vi "UI.vi"(11 "Error In":errorcluster) -> (15 "Error Out":errorcluster)   [LabVIEW 2020, in "I2C Controller.lvlib" / "I2C.lvclass"]
uses:
  I2C.lvclass
  Typedef's/I2C Timings.ctl
  Typedef's/I2C Operations.ctl
  Common/Typedef's/Protocols Queue Operations.ctl
  Common/Typedef's/Protocols Queue State.ctl
  Common/Typedef's/Protocols Event Operations.ctl
  Typedef's/I2C Data Cluster.ctl
  Parent/Protocols/Protocols.lvclass
  Parent/Protocols/Typedef's/DVR Operations.ctl
  I2C.lvclass/I2C.ctl
  I2C Controller.lvlib
panel:
  in  "Data":u8 format="%x"
  in  "Register Address":u8 format="%x"
  in  "Device Address":u8 format="%x"
  in  "Ok":bool
  in  "Operation":T1
  in  "Timings":T2={"T hd:sta"=4000, "T su:dat"=0, "T hd:dat"=0, "T low"=0, "T high"=0, "T su:sta"=5000, "T su:sto"=5000, "T buf"=5000} {"T buf" step=1 format="%#_6f"; "T su:sto" step=1 format="%#_6f"; "T su:sta" step=1 format="%#_6f"; "T high" step=1 format="%#_6f"; "T low" step=1 format="%#_6f"; "T hd:dat" step=1 format="%#_6f"; "T su:dat" step=1 format="%#_6f"; "T hd:sta" step=1 format="%#_6f"}
  # "All init values is\nfor 100khz"
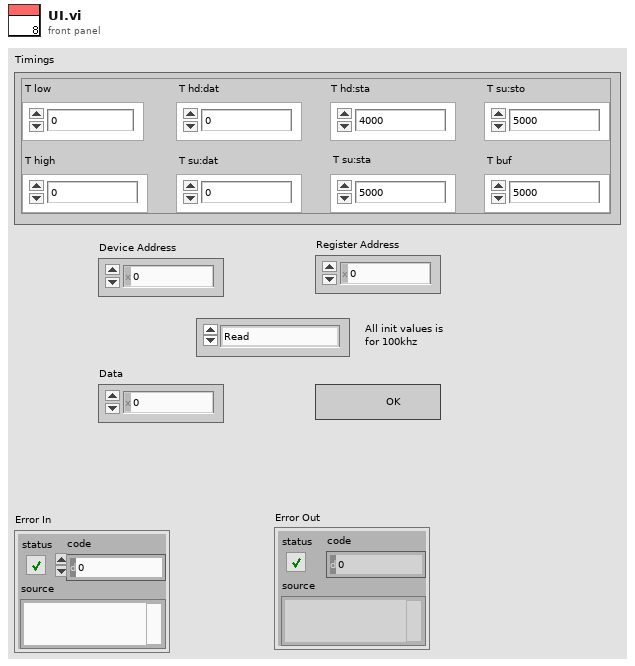
[diagram p1: front panel]
types:
  T1 = typedef "I2C Controller.lvlib/I2C.lvclass/I2C Operations.ctl" = enum16{"Read", "Write"}
  T2 = typedef "I2C Controller.lvlib/I2C.lvclass/I2C Timings.ctl" = cluster{"T hd:sta":u32, "T su:dat":u32, "T hd:dat":u32, "T low":u32, "T high":u32, "T su:sta":u32, "T su:sto":u32, "T buf":u32}
  T3 = typedef "I2C Controller.lvlib/Protocols Event Operations.ctl" = enum16{"Create", "Generate", "Destroy"}
  T4 = typedef "I2C Controller.lvlib/I2C.lvclass/I2C Data Cluster.ctl" = cluster{"Timings":T2, "Data":u8, "Operation":T1, "Device Address":u8, "Register Address":u8, "DVR Ref":refnum<data-value>, "Frequency":dbl, "Voltage":dbl}
  T5 = typedef "I2C Controller.lvlib/Protocols Queue Operations.ctl" = enum16{"Create", "Enqueue", "Dequeue", "Enstack", "Flush", "Destroy"}
  T6 = typedef "I2C Controller.lvlib/Protocols Queue State.ctl" = cluster{"State":string, "Data":variant}
  T7 = typedef "I2C Controller.lvlib/Protocols.lvclass/DVR Operations.ctl" = enum16{"Create", "Destroy"}
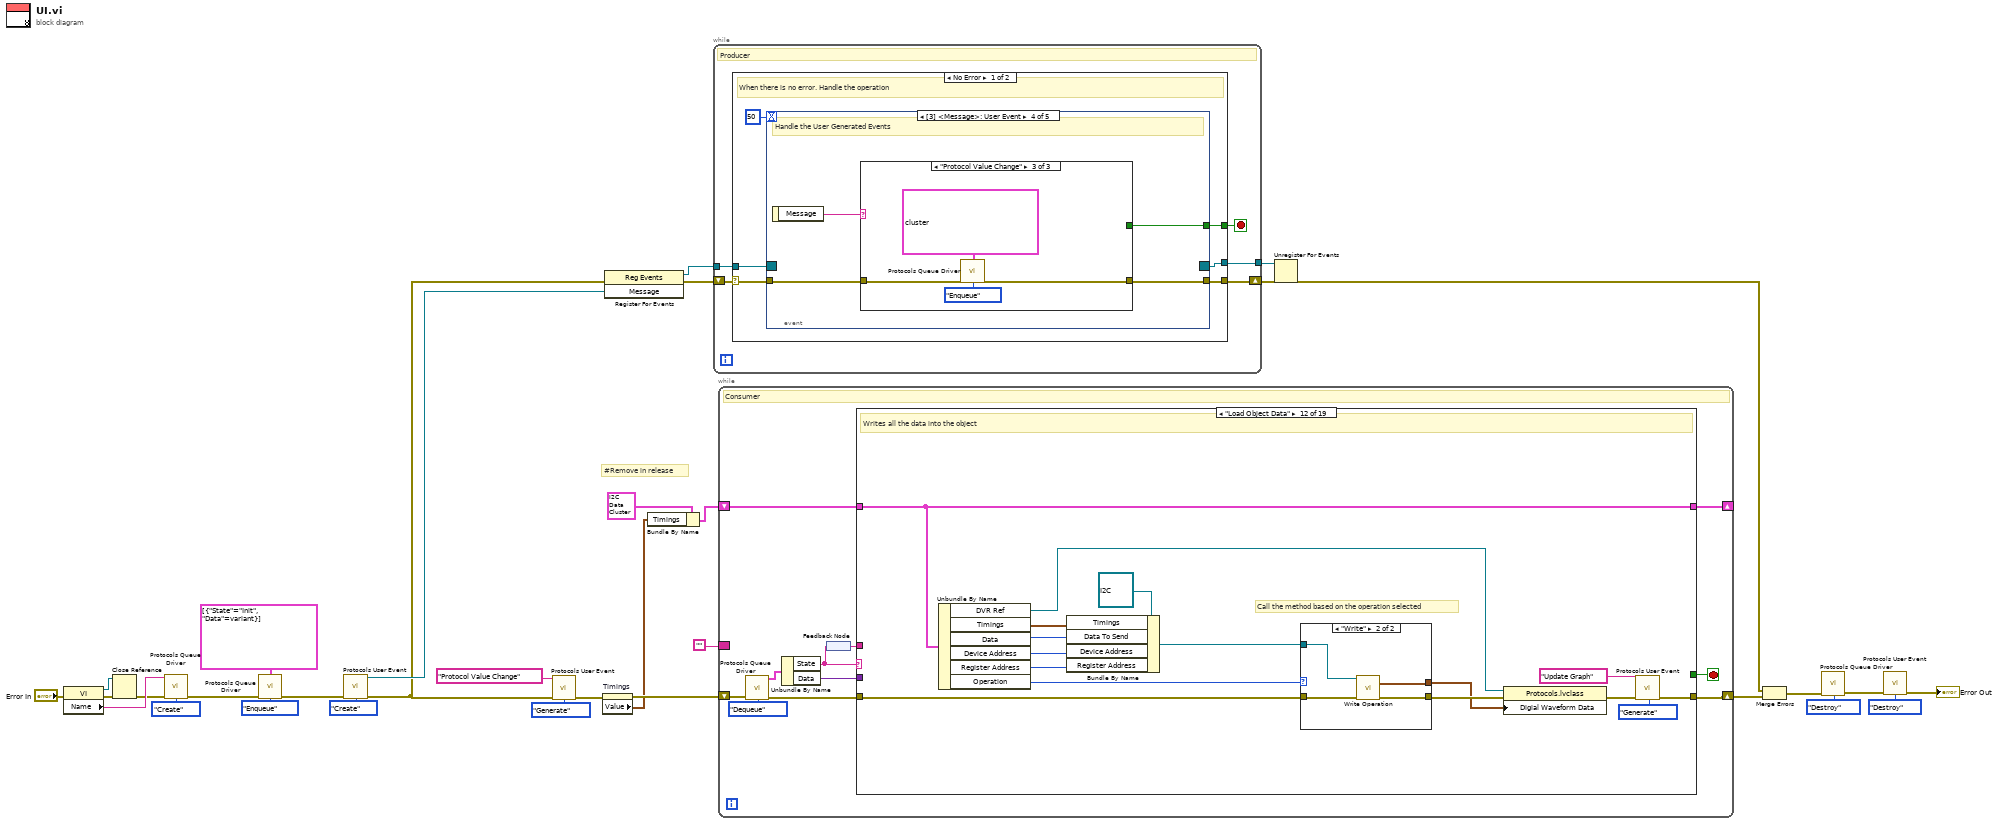
[diagram p0: block diagram]
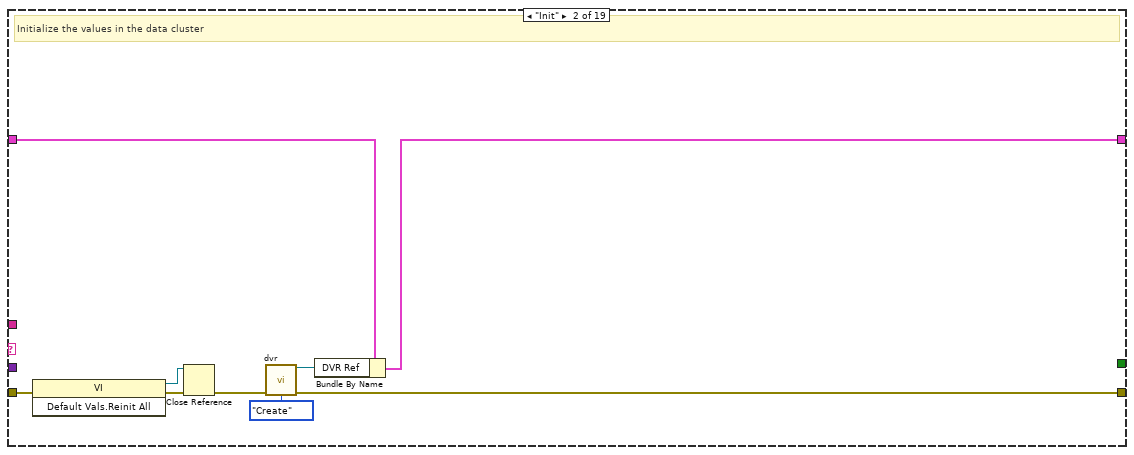
[diagram p3: hidden frame]
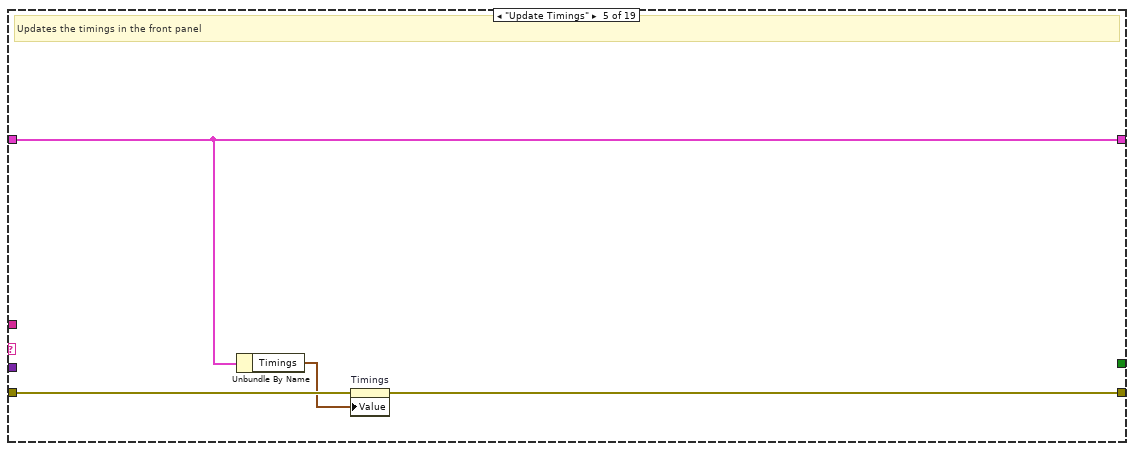
[diagram p6: hidden frame]
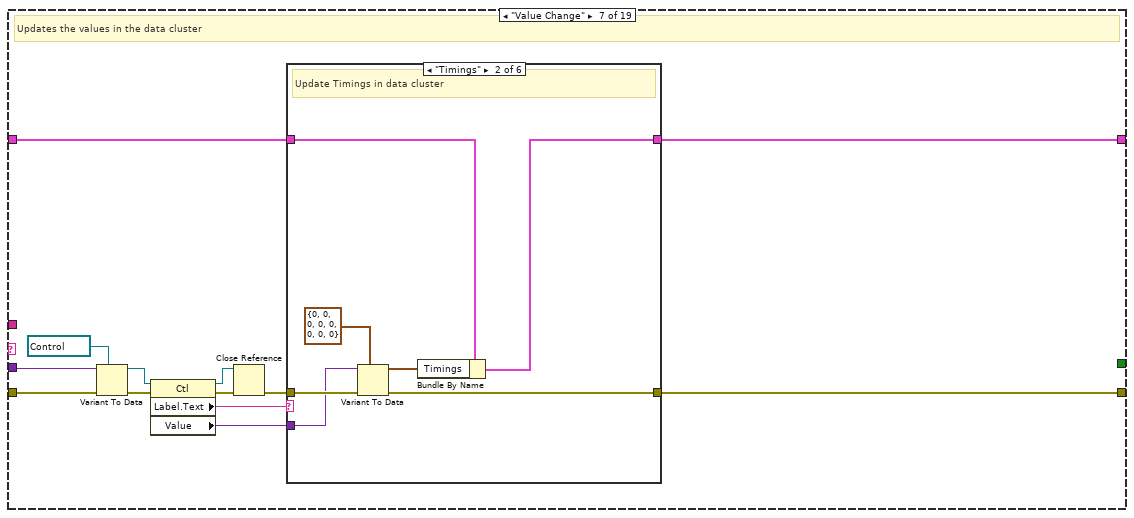
[diagram p8: hidden frame]
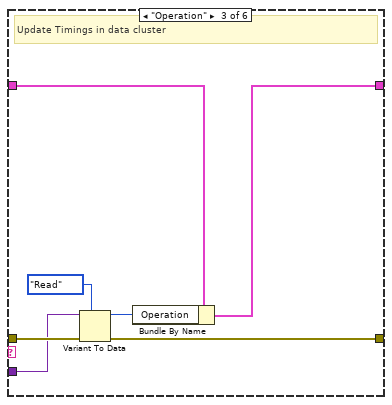
[diagram p10: hidden frame]
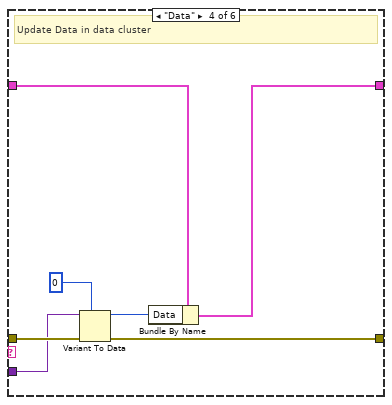
[diagram p11: hidden frame]
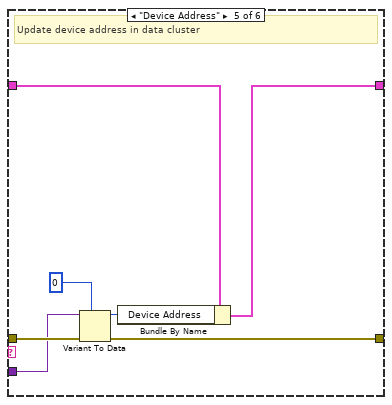
[diagram p12: hidden frame]
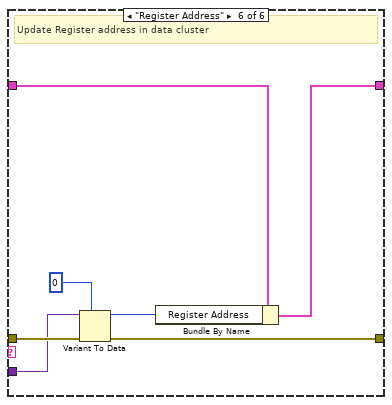
[diagram p13: hidden frame]
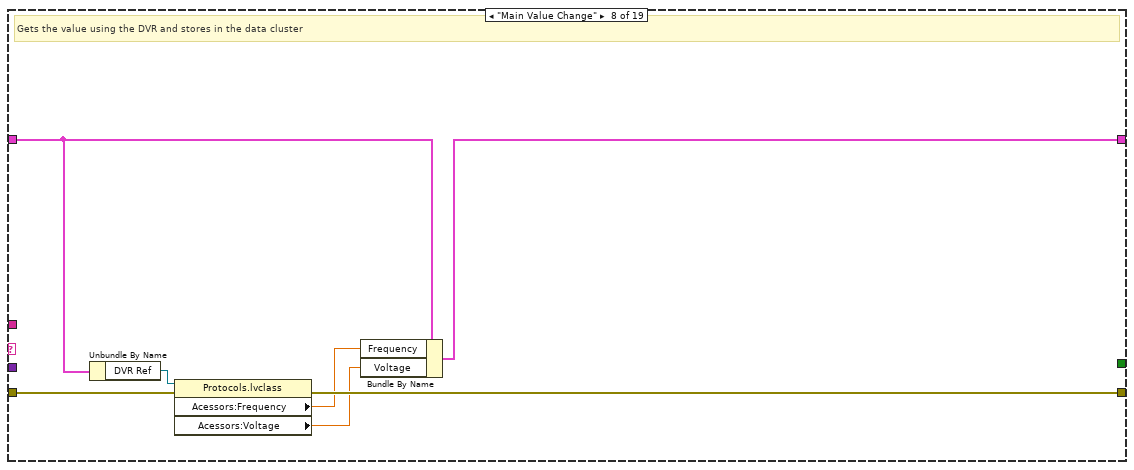
[diagram p14: hidden frame]
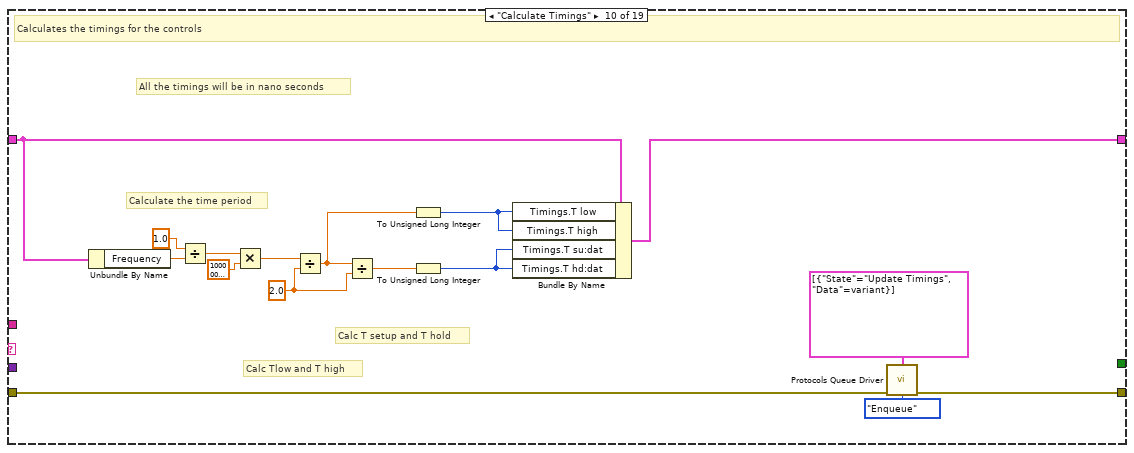
[diagram p16: hidden frame]
diagram:
  # "#Remove in release"
  n1 = property class="VI"(error in="Error In") -> (reference out=w17:refnum<vi>, error out=w15:errorcluster, "Name"=w18:string)  [unwired: 1 in]
  n2 = Close Reference(reference=w17, error in (no error)=w15) -> (error out=w16:errorcluster)
  n3 = call "Protocols Queue Driver.vi"("Queue Name"=w18, "Error In"=w16, "Q Operations"=Protocols_Queue_Operations."Create") -> ("Error Out"=w19:errorcluster)  [unwired: 11 in, 1 out]
  n4 = call "Protocols Queue Driver.vi"("State[]"=T6[] [{"State"="Init", "Data"=variant}], "Error In"=w19, "Q Operations"=Protocols_Queue_Operations."Enqueue") -> ("Error Out"=w20:errorcluster)  [unwired: 11 in, 1 out]
  n5 = call "Protocols User Event.vi"("Error In"=w20, "Enum"=Protocols_Event_Operations."Create") -> ("Message"=w24:refnum<user-event>, "Error Out"=w2:errorcluster)  [unwired: 12 in]
  n6 = call "Protocols User Event.vi"("Event Data"="Protocol Value Change", "Error In"=w2, "Enum"=Protocols_Event_Operations."Generate") -> ("Error Out"=w1:errorcluster)  [unwired: 11 in, 1 out]
  n7 = property on="Timings" class="Clust (strict)"(error in=w1) -> (error out=w7:errorcluster, "Value"=w5:T2)  [unwired: 1 in, 1 out]
  n8 = register-events(error in=w2, w24) -> (reference out=w25:refnum<event-registration>, error out=w23:errorcluster)  [unwired: 1 in]
  n9 = Bundle By Name(cluster=T4 {"Timings"={"T hd:sta"=0, "T su:dat"=0, "T hd:dat"=0, "T low"=0, "T high"=0, "T su:sta"=0, "T su:sto"=0, "T buf"=0}, "Data"=0, "Operation"=enum."Read", "Device Address"=0, "Register Address"=0, "DVR Ref"=refnum, "Frequency"=0.0, "Voltage"=0.0} ("I2C Data Cluster"), "Timings"=w5) -> (w6:T4)
  n10 = while {
    shift-right: [w36] -> w12
    shift-left: w23 -> [w37]
    tunnel: w25 -> [w35]
    tunnel: [w34] -> w27
    stop <- w33 stop-if-true
    # "Producer"
    n11 = case shown="No Error" w37 {
      selector: w37 -> [w43 w81]
      tunnel: [w42 w84] -> w36
      tunnel: w35 -> [w40 _]
      tunnel: [w39 _] -> w34
      tunnel: [w38 _] -> w33
      frame No Error {
        # "When there is no error. Handle the operation"
        n12 = event shown="[3] <Message>: User Event" {
          selector: w40 -> [_ _ _ _ _]
          dyn-events: [_ _ _ _ _] -> w39
          timeout: 50 -> [_ _ _ _ _]
          tunnel: [w44 w52 w56 w59 w75] -> w42
          tunnel: w43 -> [w44 w53 w56 w60 w74]
          tunnel: [_ _ _ w61 _] -> w38
          event Timeout {
            # "Do nothing"
            n13 = event-data() -> ()  [unwired: 1 in, 1 out]
          }
          event "Data", "Device Address", "Register Address": Value Change {
            # "Value change has occured update in data cluster"
            n14 = event-data() -> ("CtlRef"=w48:refnum<vi>)  [unwired: 1 in]
            n15 = To Variant(anything=w48) -> (Variant=w47:variant)
            n16 = Bundle By Name(cluster=T6 {"State"="", "Data"=variant} ("Dequeued State"), "State"="Value Change", "Data"=w47) -> (w46:T6)
            n17 = Initialize Array(w46, 1 ("dimension size")) -> (w45:T6[])
            n18 = call "Protocols Queue Driver.vi"("State[]"=w45, "Error In"=w53, "Q Operations"=Protocols_Queue_Operations."Enqueue") -> ("Error Out"=w52:errorcluster)  [unwired: 11 in, 1 out]
          }
          event Panel Close? {
            # "Enqueue the exit operation for panel close"
            n19 = event-data() -> ()  [unwired: 1 in, 4 out]
            n20 = call "Protocols Queue Driver.vi"("State[]"=T6[] [{"State"="Exit", "Data"=variant}], "Error In"=w56, "Q Operations"=Protocols_Queue_Operations."Enqueue") -> ()  [unwired: 11 in, 2 out]
            n21 = event-data("Discard?"=TRUE) -> ()  [unwired: 1 in, 1 out]
          }
          event User Event {
            # "Handle the User Generated Events"
            n22 = event-data() -> ("Message"=w62:string)  [unwired: 1 in]
            n23 = case shown="\"Protocol Value Change\"" w62 {
              tunnel: [_ TRUE _] -> w61
              tunnel: [w63 w64 w69] -> w59
              tunnel: w60 -> [w63 w65 w70]
              frame Default {
              }
              frame "Stop All" {
                n24 = call "Protocols Queue Driver.vi"("State[]"=T6[] [{"State"="Exit", "Data"=variant}], "Error In"=w65, "Q Operations"=Protocols_Queue_Operations."Enqueue") -> ("Error Out"=w64:errorcluster)  [unwired: 11 in, 1 out]
              }
              frame "Protocol Value Change" {
                n25 = call "Protocols Queue Driver.vi"("State[]"=T6[] [{"State"="Main Value Change", "Data"=variant}, {"State"="Calculate Timings", "Data"=variant}], "Error In"=w70, "Q Operations"=Protocols_Queue_Operations."Enqueue") -> ("Error Out"=w69:errorcluster)  [unwired: 11 in, 1 out]
              }
            }
          }
          event "Ok": Value Change {
            # "When OK Button is pressed Calculate the output"
            n26 = event-data() -> ()  [unwired: 1 in, 1 out]
            n27 = call "Protocols Queue Driver.vi"("State[]"=T6[] [{"State"="Load Object Data", "Data"=variant}, {"State"="Calculate Output", "Data"=variant}], "Error In"=w74, "Q Operations"=Protocols_Queue_Operations."Enqueue") -> ("Error Out"=w75:errorcluster)  [unwired: 11 in, 1 out]
          }
        }
      }
      frame Error {
        # "When there is error. Enqueue the error state"
        n28 = call <vilib>:"Clear Errors.vi"("error in (no error)"=w81) -> ("error out"=w85:errorcluster)  [unwired: 5 in, 1 out]
        n29 = To Variant(anything=w81) -> (Variant=w80:variant)
        n30 = Bundle By Name(cluster=T6 {"State"="", "Data"=variant} ("Dequeued State"), "State"="Producer Error", "Data"=w80) -> (w79:T6)
        n31 = Initialize Array(w79, 1 ("dimension size")) -> (w78:T6[])
        n32 = call "Protocols Queue Driver.vi"("State[]"=w78, "Error In"=w85, "Q Operations"=Protocols_Queue_Operations."Enqueue") -> ("Error Out"=w84:errorcluster)  [unwired: 11 in, 1 out]
      }
    }
  }
  n33 = while {
    shift-right: [w93] -> w11
    shift-left: w7 -> [w96]
    border: "" -> [_]
    shift-right: [w87] -> _
    shift-left: w6 -> [w88]
    stop <- w91 stop-if-true
    # "Consumer"
    n34 = call "Protocols Queue Driver.vi"("Error In"=w96, "Q Operations"=Protocols_Queue_Operations."Dequeue") -> ("Dequeued State"=w95:T6, "Error Out"=w94:errorcluster)  [unwired: 12 in]
    n35 = Unbundle By Name(w95) -> ("State"=w90:string, "Data"=w92:variant)
    n36 = feedback-in #1(w90) -> ()
    n37 = feedback #1() -> (w89:string)
    n38 = case shown="\"Load Object Data\"" w90 {
      tunnel: w94 -> [w99 w108 w110 w112 w116 w118 w131 w175 w177 w179 w195 w204 w218 w220 w232 w241 w261 w269 w274]
      tunnel: [w99 w103 w110 w112 w115 w118 w123 w173 w177 w178 w195 w197 w218 w220 w223 w245 w260 w269 w273] -> w93
      tunnel: w92 -> [_ _ _ _ _ _ w129 _ _ _ _ _ _ _ _ w242 _ _ _]
      tunnel: [_ _ _ _ _ _ _ _ _ _ _ _ _ _ _ _ _ _ TRUE] -> w91
      tunnel: w89 -> [_ _ _ _ _ _ _ _ _ _ _ _ _ _ w228 _ w262 _ _]
      tunnel: w88 -> [w98 w107 w109 w111 w113 w117 w120 w174 w176 w189 w194 w210 w217 w219 w221 w239 w258 w268 w270]
      tunnel: [w98 w101 w109 w111 w113 w117 w119 w171 w176 w188 w194 w210 w217 w219 w221 w239 w258 w268 w270] -> w87
      frame "/**** Initialization ****/" {
      }
      frame "Init" {
        # "Initialize the values in the data cluster"
        n39 = invoke class="VI" method="Default Vals.Reinit All"(error in=w108) -> (reference out=w104:refnum<vi>, error out=w106:errorcluster)  [unwired: 2 in, 1 out]
        n40 = Close Reference(reference=w104, error in (no error)=w106) -> (error out=w105:errorcluster)
        n41 = call "dvr.vi"("Error In"=w105, "DVR Operation"=DVR_Operations."Create") -> ("DVR Ref"=w100:refnum<data-value>, "Error Out"=w103:errorcluster)  [unwired: 12 in]
        n42 = Bundle By Name(cluster=w107, "DVR Ref"=w100) -> (w101:T4)
      }
      frame "/**** FP Related *****/" {
      }
      frame "FP Update" {
        # "Update the front panel controls"
      }
      frame "Update Timings" {
        # "Updates the timings in the front panel"
        n43 = Unbundle By Name(w113) -> ("Timings"=w114:T2)
        n44 = property on="Timings" class="Clust (strict)"(error in=w116, "Value"=w114) -> (error out=w115:errorcluster)  [unwired: 1 in, 1 out]
      }
      frame "/**** Value Change ****/" {
      }
      frame "Value Change" {
        # "Updates the values in the data cluster"
        n45 = Variant To Data(error in=w131, type=refnum<vi> refnum ("CtlRef"), Variant=w129) -> (data=w126:refnum<vi>, error out=w130:errorcluster)
        n46 = property class="Ctl"(reference=w126, error in=w130) -> (reference out=w124:refnum<vi>, error out=w127:errorcluster, "Label.Text"=w121:string, "Value"=w122:variant)
        n47 = Close Reference(reference=w124, error in (no error)=w127) -> (error out=w125:errorcluster)
        n48 = case shown="\"Timings\"" w121 {
          tunnel: w125 -> [w133 w140 w147 w154 w161 w168]
          tunnel: [w133 w137 w144 w151 w158 w165] -> w123
          tunnel: w122 -> [_ w136 w143 w150 w157 w164]
          tunnel: [w132 w138 w145 w152 w159 w166] -> w119
          tunnel: w120 -> [w132 w139 w146 w153 w160 w167]
          frame Default {
            # "When the control name mismatches"
          }
          frame "Timings" {
            # "Update Timings in data cluster"
            n49 = Variant To Data(error in=w140, type=T2 {"T hd:sta"=0, "T su:dat"=0, "T hd:dat"=0, "T low"=0, "T high"=0, "T su:sta"=0, "T su:sto"=0, "T buf"=0} ("Timings"), Variant=w136) -> (data=w134:T2, error out=w137:errorcluster)
            n50 = Bundle By Name(cluster=w139, "Timings"=w134) -> (w138:T4)
          }
          frame "Operation" {
            # "Update Timings in data cluster"
            n51 = Variant To Data(error in=w147, type=I2C_Operations."Read" ("Operation"), Variant=w143) -> (data=w142:T1, error out=w144:errorcluster)
            n52 = Bundle By Name(cluster=w146, "Operation"=w142) -> (w145:T4)
          }
          frame "Data" {
            # "Update Data in data cluster"
            n53 = Variant To Data(error in=w154, type=u8 0 ("Data"), Variant=w150) -> (data=w149:u8, error out=w151:errorcluster)
            n54 = Bundle By Name(cluster=w153, "Data"=w149) -> (w152:T4)
          }
          frame "Device Address" {
            # "Update device address in data cluster"
            n55 = Variant To Data(error in=w161, type=u8 0 ("Data"), Variant=w157) -> (data=w156:u8, error out=w158:errorcluster)
            n56 = Bundle By Name(cluster=w160, "Device Address"=w156) -> (w159:T4)
          }
          frame "Register Address" {
            # "Update Register address in data cluster"
            n57 = Variant To Data(error in=w168, type=u8 0 ("Data"), Variant=w164) -> (data=w163:u8, error out=w165:errorcluster)
            n58 = Bundle By Name(cluster=w167, "Register Address"=w163) -> (w166:T4)
          }
        }
      }
      frame "Main Value Change" {
        # "Gets the value using the DVR and stores in the data cluster"
        n59 = Unbundle By Name(w174) -> ("DVR Ref"=w172:refnum<data-value>)
        n60 = property class="Protocols.lvclass"(reference=w172, error in=w175) -> (error out=w173:errorcluster, "Acessors:Frequency"=w170:dbl, "Acessors:Voltage"=w169:dbl)  [unwired: 1 out]
        n61 = Bundle By Name(cluster=w174, "Frequency"=w170, "Voltage"=w169) -> (w171:T4)
      }
      frame "/***** functionalities ****/" {
      }
      frame "Calculate Timings" {
        w190 = 2.0 ("y")
        # "All the timings will be in nano seconds"
        # "Calc T setup and T hold"
        # "Calc Tlow and T high"
        # "Calculate the time period"
        # "Calculates the timings for the controls"
        n62 = Unbundle By Name(w189) -> ("Frequency"=w193:dbl)
        n63 = Divide(x=1.0 ("y"), y=w193) -> (x/y=w191:dbl)
        n64 = Multiply(x=w191, y=1000000000.0) -> (x*y=w185:dbl)
        n65 = Divide(x=w185, y=w190) -> (x/y=w186:dbl)
        n66 = Divide(x=w186, y=w190) -> (x/y=w183:dbl)
        n67 = To Unsigned Long Integer(number=w186) -> (unsigned 32bit integer=w184:u32)
        n68 = To Unsigned Long Integer(number=w183) -> (unsigned 32bit integer=w182:u32)
        n69 = Bundle By Name(cluster=w189, "Timings.T low"=w184, "Timings.T high"=w184, "Timings.T su:dat"=w182, "Timings.T hd:dat"=w182) -> (w188:T4)
        n70 = call "Protocols Queue Driver.vi"("State[]"=T6[] [{"State"="Update Timings", "Data"=variant}], "Error In"=w179, "Q Operations"=Protocols_Queue_Operations."Enqueue") -> ("Error Out"=w178:errorcluster)  [unwired: 11 in, 1 out]
      }
      frame "" {
        # "Do nothing"
      }
      frame "Load Object Data" {
        # "Call the method based on the operation selected"
        # "Writes all the data into the object"
        n71 = Unbundle By Name(w210) -> ("DVR Ref"=w201:refnum<data-value>, "Timings"=w209:T2, "Data"=w206:u8, "Device Address"=w208:u8, "Register Address"=w207:u8, "Operation"=w203:T1)
        n72 = Bundle By Name(cluster=refnum<class "I2C.lvclass"> refnum ("I2C Controller.lvlib:I2C.lvclass"), "Timings"=w209, "Data To Send"=w206, "Device Address"=w208, "Register Address"=w207) -> (w202:refnum<class "I2C.lvclass">)
        n73 = case shown="\"Write\"" w203 {
          tunnel: [w212 w216] -> w205
          tunnel: w204 -> [w212 w215]
          tunnel: w202 -> [_ w214]
          tunnel: [_ w213] -> w200
          frame "Read", Default {
          }
          frame "Write" {
            n74 = call-dynamic "Write Operation.vi"("I2C in"=w214, "Error In"=w215) -> ("Digial Waveform Data"=w213:digitalwaveform, "Error Out"=w216:errorcluster)  [unwired: 11 in, 1 out]
          }
        }
        n75 = property class="Protocols.lvclass"(reference=w201, error in=w205, "Digial Waveform Data"=w200) -> (error out=w198:errorcluster)  [unwired: 1 out]
        n76 = call "Protocols User Event.vi"("Event Data"="Update Graph", "Error In"=w198, "Enum"=Protocols_Event_Operations."Generate") -> ("Error Out"=w197:errorcluster)  [unwired: 11 in, 1 out]
      }
      frame "Calculate Output" {
        # "Performs the operation and send the data to the main VI"
      }
      frame "/***** Error States ****/" {
      }
      frame "Error" {
        # "Handle the error"
        n77 = Unbundle By Name(w232) -> ("code"=w230:i32, "source"=w229:string)
        n78 = call <vilib>:"Clear Errors.vi"("error in (no error)"=w232) -> ("error out"=w233:errorcluster)  [unwired: 5 in, 1 out]
        n79 = Format Into String(format string="Erorr Occured in State : %s !!!\nError Code : %d\nError Description : %s", error in=w233, w228, w230, w229) -> (resulting string=w227:string, error out=w224:errorcluster)  [unwired: 1 in]
        n80 = Two Button Dialog(message=w227, 1:"Stop" ("F button name (\"Cancel\")"), 2:"Continue" ("T button name (\"OK\")")) -> (T button?=w222:bool)
        n81 = case shown="True" w222 {
          tunnel: w224 -> [w236 w238]
          tunnel: [w235 w238] -> w223
          frame False {
            n82 = call "Protocols Queue Driver.vi"("State[]"=T6[] [{"State"="Exit", "Data"=variant}], "Error In"=w236, "Q Operations"=Protocols_Queue_Operations."Enqueue") -> ("Error Out"=w235:errorcluster)  [unwired: 11 in, 1 out]
          }
          frame True {
          }
        }
      }
      frame "Producer Error" {
        # "Handle the producer error"
        n83 = Variant To Data(error in=w241, type=w241, Variant=w242) -> (data=w240:errorcluster, error out=w243:errorcluster)
        n84 = Unbundle By Name(w240) -> ("code"=w251:i32, "source"=w250:string)
        n85 = Format Into String(format string="Erorr Occured in Producer !!!\nError Code : %d\nError Description : %s", error in=w243, w251, w250) -> (resulting string=w249:string, error out=w246:errorcluster)  [unwired: 1 in]
        n86 = Two Button Dialog(message=w249, 1:"Stop" ("F button name (\"Cancel\")"), 2:"Continue" ("T button name (\"OK\")")) -> (T button?=w244:bool)
        n87 = case shown="True" w244 {
          tunnel: w246 -> [w255 w257]
          tunnel: [w254 w257] -> w245
          frame False {
            n88 = call "Protocols Queue Driver.vi"("State[]"=T6[] [{"State"="Exit", "Data"=variant}], "Error In"=w255, "Q Operations"=Protocols_Queue_Operations."Enqueue") -> ("Error Out"=w254:errorcluster)  [unwired: 11 in, 1 out]
          }
          frame True {
          }
        }
      }
      frame "Developer Error", Default {
        n89 = One Button Dialog(message=w262) -> (true=w259:bool)  [unwired: 1 in]
        n90 = case shown="True" w259 {
          tunnel: w261 -> [w263 w266]
          tunnel: [w263 w265] -> w260
          frame False {
          }
          frame True {
            n91 = call "Protocols Queue Driver.vi"("State[]"=T6[] [{"State"="Exit", "Data"=variant}], "Error In"=w266, "Q Operations"=Protocols_Queue_Operations."Enqueue") -> ("Error Out"=w265:errorcluster)  [unwired: 11 in, 1 out]
          }
        }
      }
      frame "/***** Exit States ****/" {
      }
      frame "Exit" {
        # "Stop all the operation and exit"
        n92 = call "Protocols User Event.vi"("Event Data"="Stop All", "Error In"=w274, "Enum"=Protocols_Event_Operations."Generate") -> ("Error Out"=w273:errorcluster)  [unwired: 11 in, 1 out]
      }
    }
  }
  n93 = Unregister For Events(event registration refnum=w27, error in=w12) -> (error out=w26:errorcluster)
  n94 = Merge Errors(w26, w11) -> (w30:errorcluster)
  n95 = call "Protocols Queue Driver.vi"("Error In"=w30, "Q Operations"=Protocols_Queue_Operations."Destroy") -> ("Error Out"=w31:errorcluster)  [unwired: 12 in, 1 out]
  n96 = call "Protocols User Event.vi"("Error In"=w31, "Enum"=Protocols_Event_Operations."Destroy") -> ("Error Out"=→"Error Out":errorcluster)  [unwired: 12 in, 1 out]
